vi "Wait If Occupied.vi"(8 "Replication Square":refnum<class "Square.lvclass">, 9 "Direction":T3, 10 "Action if Empty":T2, 11 "Square In":refnum<class "Square.lvclass">) -> (3 "Run Result":T1)   [LabVIEW 2020, in "SquareBattle.lvlib"]
uses:
  SquareBattle.lvlib
  Action.ctl
  Direction.ctl
  Run Result.ctl
  Square/Square.lvclass
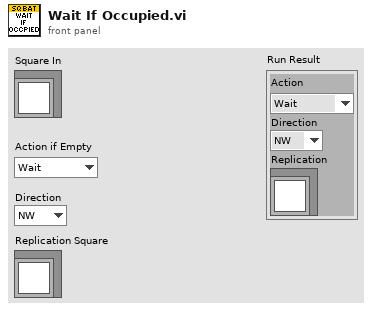
[diagram p1: front panel]
types:
  T1 = typedef "SquareBattle.lvlib/Run Result.ctl" = cluster{"Action":T2, "Direction":T3, "Replication":refnum<class "Square.lvclass">}
  T2 = typedef "SquareBattle.lvlib/Action.ctl" = enum16{"Wait", "Move", "Attack", "Replicate"}
  T3 = typedef "SquareBattle.lvlib/Direction.ctl" = enum16{"NW", "N", "NE", "E", "SE", "S", "SW", "W"}
  T4 = typedef "SquareBattle.lvlib/Location Status.ctl" = cluster{"Empty":bool, "Friend":bool, "Enemy":bool}
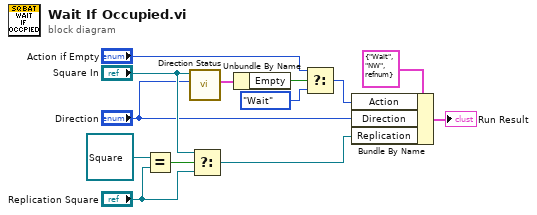
[diagram p0: block diagram]
diagram:
  n1 = Equal?(x=refnum<class "Square.lvclass"> refnum, y="Replication Square") -> (x = y?=w11:bool)
  n2 = call "Direction Status.vi"("Direction"="Direction", "Square"="Square In") -> ("Status"=w8:T4)  [unwired: 9 in]
  n3 = Select(t="Square In", s=w11, f="Replication Square") -> (s? t:f=w1:refnum<class "Square.lvclass">)
  n4 = Unbundle By Name(w8) -> ("Empty"=w7:bool)
  n5 = Select(t="Action if Empty", s=w7, f=Action."Wait") -> (s? t:f=w2:T2)
  n6 = Bundle By Name(cluster=T1 {"Action"=enum."Wait", "Direction"=enum."NW", "Replication"=refnum} ("Run Result"), "Action"=w2, "Direction"="Direction", "Replication"=w1) -> (→"Run Result":T1)
